vi "Set-external-timing-status.vi"(8 "error in":errorcluster, 9 "Reset errors?":bool, 10 "Timing status in":T1=enum."Active", 11 "Data ref. in":refnum<data-value>) -> (0 "error IO":errorcluster, 2 "Timing status":T1, 3 "Data ref.":refnum<data-value>)   [LabVIEW 2013, in "CameraVision.lvlib" / "CV-Main.lvclass"]
doc: "This function loads the default values for the hidden program parameters from an .xml file and writes these values to the parameter groups.\nThe file path for the hidden parameters is '<Application directory>\\Program data\\parameters-hidden.xml'.\nThe hidden parameters can not be changed through the CameraVision program, but can be changed using the 'CV-Set-hidden-parameters.vi' utility."
uses:
  CV-Main.lvclass
  UI/Module-states.ctl
  CV-Main.lvclass/CV-Main.ctl
  Configuration/CV-Configuration.lvclass/CV-Configuration.ctl
  Read Config params.vi
  Configuration/Read Timing status.vi
  Configuration/Write Timing status.vi
  Configuration/CV-Configuration.lvclass
  UI/CV-UI.lvclass
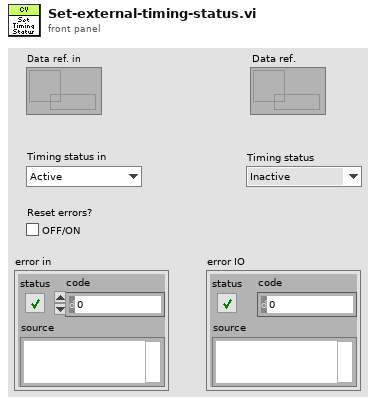
[diagram p1: front panel]
types:
  T1 = typedef "CameraVision.lvlib/CV-UI.lvclass/Module-states.ctl" = enum16{"Inactive", "Active", "Data-loss", "Error", "Simulation", "Synchronizing", "Initialized", "Released"}
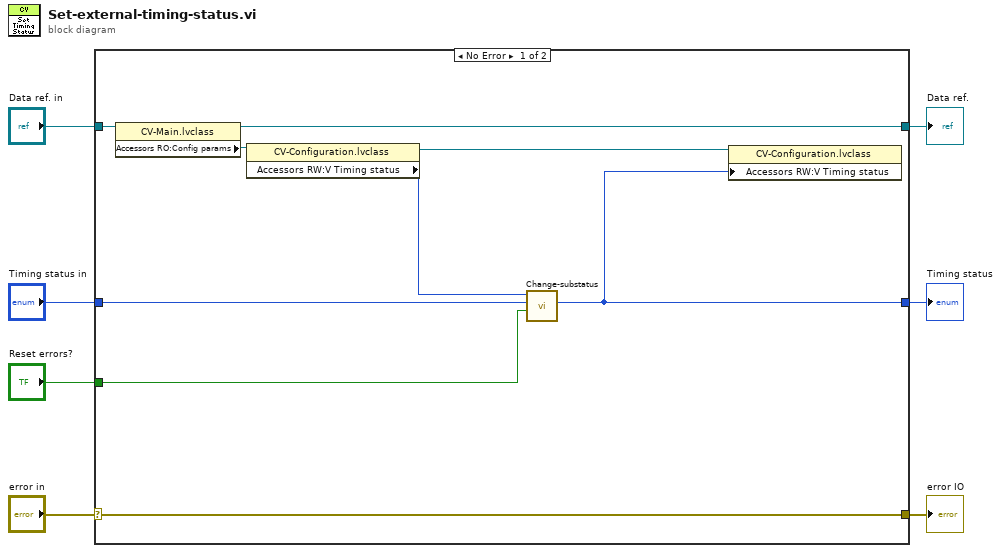
[diagram p0: block diagram]
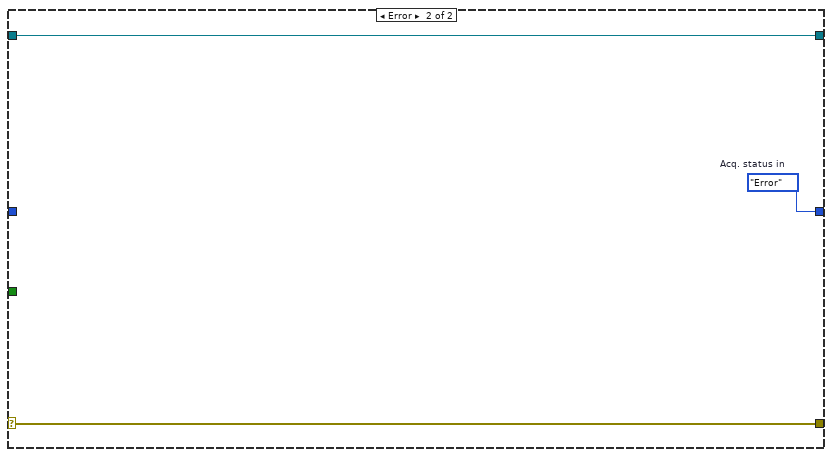
[diagram p2: hidden frame]
diagram:
  n1 = case shown="No Error" "error in" {
    selector: "error in" -> [w10 w19]
    tunnel: [w10 w19] -> w7
    tunnel: "Data ref. in" -> [w16 w18]
    tunnel: [w15 w18] -> w4
    tunnel: "Timing status in" -> [w11 _]
    tunnel: "Reset errors?" -> [w13 _]
    tunnel: [w8 w17] -> w1
    frame No Error {
      n2 = property class="CV-Main.lvclass"(reference=w16) -> (reference out=w15:refnum<data-value>, "Accessors RO:Config params"=w14:refnum<data-value>)  [unwired: 1 in, 1 out]
      n3 = property class="CV-Configuration.lvclass"(reference=w14) -> (reference out=w9:refnum<data-value>, "Accessors RW:V Timing status"=w12:T1)  [unwired: 1 in, 1 out]
      n4 = call "Change-substatus.vi"("Reset errors?"=w13, "New status in"=w11, "Previous status"=w12) -> ("New status"=w8:T1)  [unwired: 8 in]
      n5 = property class="CV-Configuration.lvclass"(reference=w9, "Accessors RW:V Timing status"=w8) -> ()  [unwired: 1 in, 2 out]
    }
    frame Error {
      w17 = Module-states."Error"  # Acq. status in
    }
  }
  "error IO" <- w7
  "Data ref." <- w4
  "Timing status" <- w1
